vi "Delete RF Connection.vi"(8 "error in (no error)":errorcluster, 10 "RF Connection (\"RF1.1\")":string="RF1.1", 11 "VISA resource name":refnum<visa-resource-name>) -> (0 "error out":errorcluster, 3 "VISA resource name out":refnum<visa-resource-name>)   [LabVIEW 2015, in "Rohde&Schwarz CMXP Base.lvlib"]
doc: "Deletes a signal path.\n\nAttribute:\nRSCMXPBASE_ATTR_RF_CONNECTION_DELETE\n\nRemote-control command:\nDELete:TENVironment:SPATh"
uses:
  <instrlib>/Rohde&Schwarz CMXP Base/Rohde&Schwarz CMXP Base.lvlib
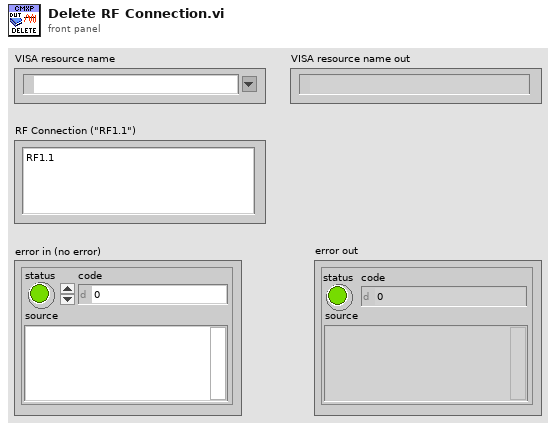
[diagram p1: front panel]
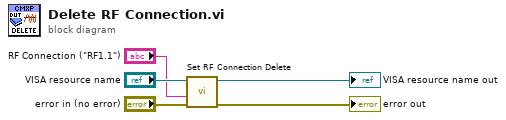
[diagram p0: block diagram]
diagram:
  n1 = call "Set RF Connection Delete"("error in (no error)"="error in (no error)", "RF Connection Delete ()"="RF Connection (\"RF1.1\")", "instrument handle"="VISA resource name") -> ("error out"=→"error out":errorcluster, "instrument handle out"=→"VISA resource name out":refnum<visa-resource-name>)  [unwired: 7 in]
